vi "DAQ Loop.vi"(8 "error in":errorcluster, 10 "Queues":T1, 11 "Notifiers":T2) -> (0 "error out":errorcluster)   [LabVIEW 2015, in "DAQ.lvlib"]
uses:
  DAQ.lvlib
  support/Message Queue/Message Queue.lvlib
  TypeDefs/DAQ data.ctl
  <vilib>/ErrorRing/Error Ring.xnode
  PLC/PLC.lvlib
  support/Global names.vi
  <vilib>/Utility/error.llb/Error Cluster From Error Code.vi
  support/Message Queue/Message Cluster.ctl
  support/Notifiers/Notifiers.ctl
  Support/Notifiers/Notifiers.lvlib
  support/Message Queue/All Message Queues.ctl
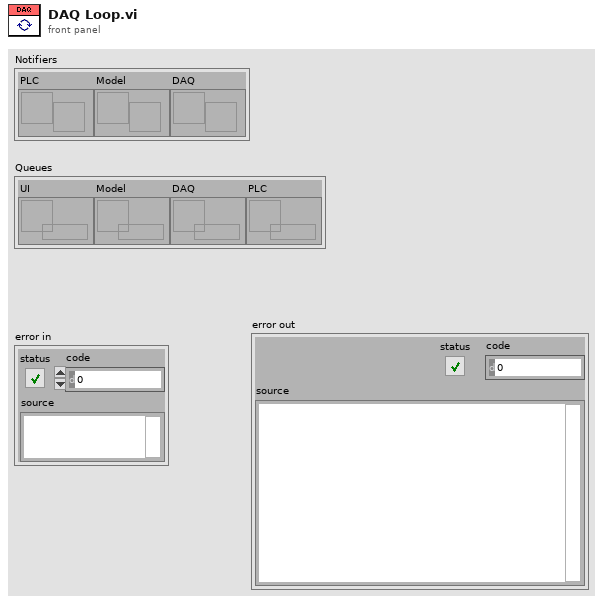
[diagram p1: front panel]
types:
  T1 = typedef "Message Queue.lvlib/All Message Queues.ctl" = cluster{"UI":refnum<queue>, "Model":refnum<queue>, "DAQ":refnum<queue>, "PLC":refnum<queue>}
  T2 = typedef "Notifiers.lvlib/Notifiers.ctl" = cluster{"PLC":refnum<notifier>, "Model":refnum<notifier>, "DAQ":refnum<notifier>}
  T3 = typedef "DAQ.lvlib/DAQ data.ctl" = cluster{"Power switch (DI)":cluster{"Channel":tag, "Data":bool}, "Dispose barrel (DI)":cluster{"Channel":tag, "Data":bool}, "Pump status (DO)":cluster{"Channel":tag, "Data":bool}, "Barrel position (AI)":cluster{"Channel":tag, "Data":dbl}}
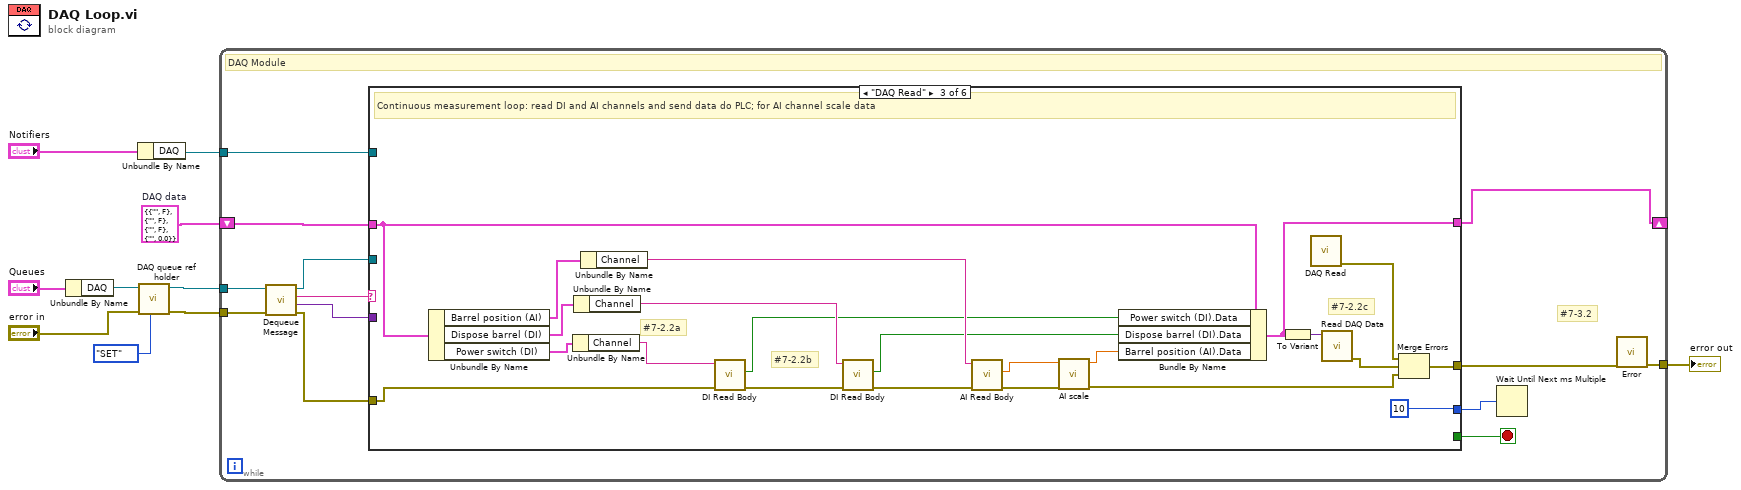
[diagram p0: block diagram]
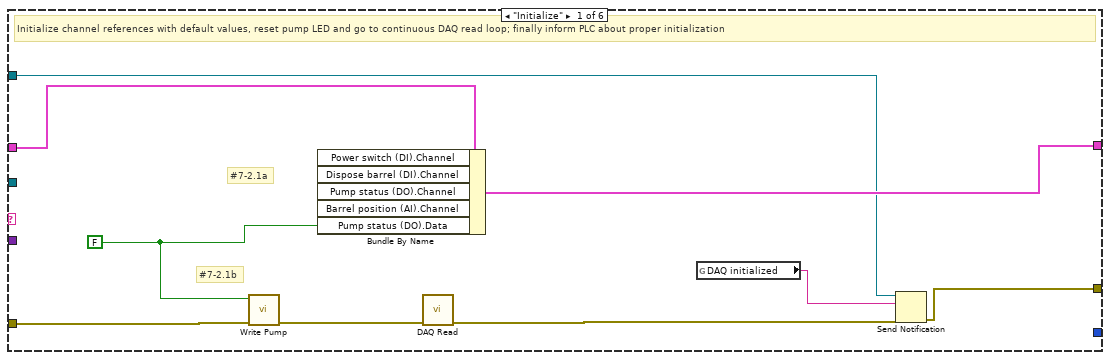
[diagram p2: hidden frame]
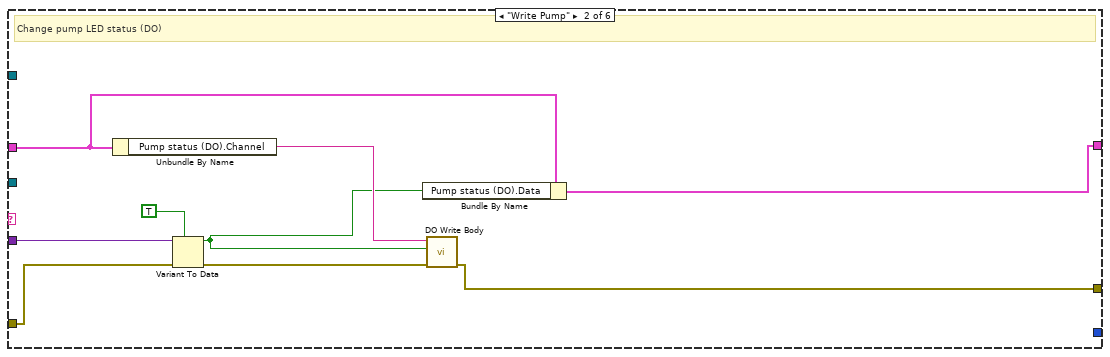
[diagram p3: hidden frame]
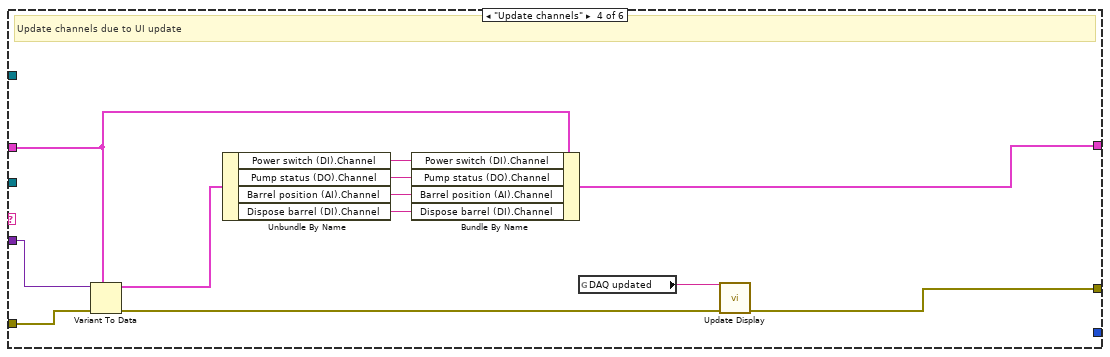
[diagram p4: hidden frame]
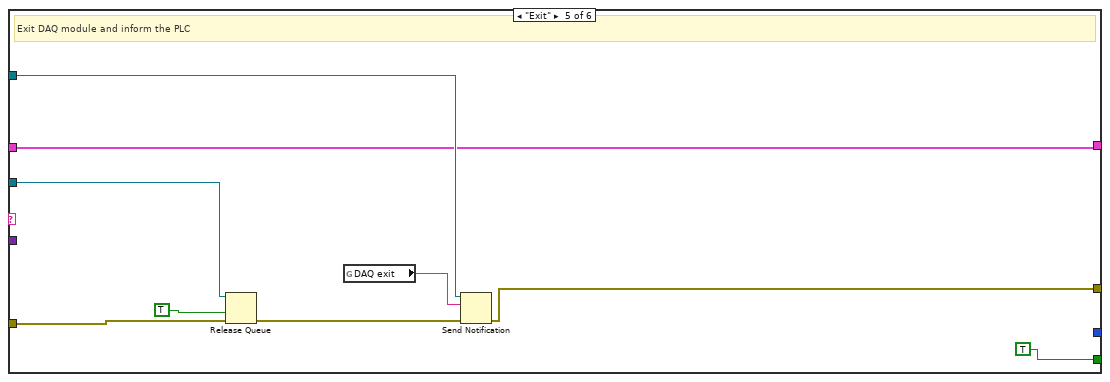
[diagram p5: hidden frame]
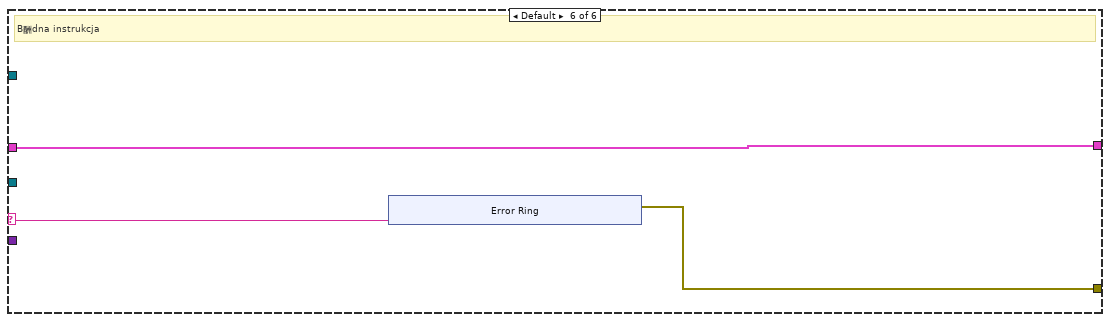
[diagram p6: hidden frame]
diagram:
  w10 = T3 {"Power switch (DI)"={"Channel"="", "Data"=FALSE}, "Dispose barrel (DI)"={"Channel"="", "Data"=FALSE}, "Pump status (DO)"={"Channel"="", "Data"=FALSE}, "Barrel position (AI)"={"Channel"="", "Data"=0.0}}  # DAQ data
  n1 = Unbundle By Name("Queues") -> ("DAQ"=w5:refnum<queue>)
  n2 = Unbundle By Name("Notifiers") -> ("DAQ"=w6:refnum<notifier>)
  n3 = call "DAQ queue ref holder.vi"("Action"=enum16{"GET", "SET"}."SET", "error in"="error in", "Message Queue In"=w5) -> ("error out"=w3:errorcluster, "Input Message Queue"=w4:refnum<queue>)  [unwired: 7 in]
  n4 = while {
    tunnel: w3 -> [w23]
    tunnel: w4 -> [w11]
    tunnel: w6 -> [w19]
    shift-right: [w18] -> _
    shift-left: w10 -> [w16]
    tunnel: [w14] -> w8
    stop <- w20 stop-if-true
    # "#7-3.2"
    # "DAQ Module"
    n5 = call "Dequeue Message.vi"("error in (no error)"=w23, "Message Queue"=w11) -> ("error out"=w22:errorcluster, "Message Data"=w21:variant, "Message"=w12:string, "dup Message Queue"=w13:refnum<queue>)  [unwired: 6 in]
    n6 = case shown="\"DAQ Read\"" w12 {
      selector: w12 -> [_ _ _ _ _ w86]
      tunnel: w22 -> [w29 w41 w56 w74 w78 _]
      tunnel: [w32 w33 w54 w66 w77 w85] -> w15
      tunnel: w21 -> [_ w40 _ w75 _ _]
      tunnel: [_ _ _ _ TRUE _] -> w20
      tunnel: w13 -> [_ _ _ _ w84 _]
      tunnel: w19 -> [w27 _ _ _ w83 _]
      tunnel: w16 -> [w31 w37 w61 w73 w79 w87]
      tunnel: [w30 w39 w58 w68 w79 w87] -> w18
      tunnel: [_ _ u32 10 ("millisecond multiple") _ _ _] -> w17
      frame "Initialize" {
        w24 = FALSE ("Pump status (DO).Data")
        # "#7-2.1b"
        # "#7-2.1a"
        # "Initialize channel references with default values, reset pump LED and go to continuous DAQ read loop; finally inform PLC about proper initialization"
        n7 = call "Write Pump.vi"("error in"=w29, "Pump state"=w24) -> ("error out"=w28:errorcluster)  [unwired: 9 in]
        n8 = Bundle By Name(cluster=w31, "Pump status (DO).Data"=w24) -> (w30:T3)  [unwired: 4 in]
        n9 = call "DAQ Read.vi"("error in"=w28) -> ("error out"=w26:errorcluster)  [unwired: 10 in]
        n10 = global read "Global names.vi" "DAQ initialized"() -> (w25:string)
        n11 = Send Notification(notification=w25, notifier=w27, error in (no error)=w26) -> (error out=w32:errorcluster)  [unwired: 1 out]
      }
      frame "Write Pump" {
        # "Change pump LED status (DO)"
        n12 = Unbundle By Name(w37) -> ("Pump status (DO).Channel"=w38:tag)
        n13 = Variant To Data(error in=w41, type=TRUE, Variant=w40) -> (data=w35:bool, error out=w34:errorcluster)
        n14 = Bundle By Name(cluster=w37, "Pump status (DO).Data"=w35) -> (w39:T3)
        n15 = call "DO Write Body.vi"("error in"=w34, "data"=w35, "Channel"=w38) -> ("error out"=w33:errorcluster)  [unwired: 6 in]
      }
      frame "DAQ Read" {
        # "#7-2.2c"
        # "#7-2.2b"
        # "#7-2.2a"
        # "Continuous measurement loop: read DI and AI channels and send data do PLC; for AI channel scale data"
        n16 = Unbundle By Name(w61) -> ("Barrel position (AI)"=w50:cluster{"Channel":tag, "Data":dbl}, "Dispose barrel (DI)"=w49:cluster{"Channel":tag, "Data":bool}, "Power switch (DI)"=w48:cluster{"Channel":tag, "Data":bool})
        n17 = Unbundle By Name(w48) -> ("Channel"=w45:tag)
        n18 = Unbundle By Name(w49) -> ("Channel"=w46:tag)
        n19 = Unbundle By Name(w50) -> ("Channel"=w47:tag)
        n20 = call "DI Read Body.vi"("error in"=w56, "Channel"=w45) -> ("error out"=w63:errorcluster, "data"=w44:bool)  [unwired: 6 in]
        n21 = call "DI Read Body.vi"("error in"=w63, "Channel"=w46) -> ("error out"=w62:errorcluster, "data"=w43:bool)  [unwired: 6 in]
        n22 = call "AI Read Body.vi"("error in"=w62, "Channel"=w47) -> ("error out"=w55:errorcluster, "data"=w51:dbl)  [unwired: 6 in]
        n23 = call "AI scale.vi"("error in"=w55, "Data in"=w51) -> ("error out"=w52:errorcluster, "Data out"=w60:dbl)  [unwired: 8 in]
        n24 = Bundle By Name(cluster=w61, "Power switch (DI).Data"=w44, "Dispose barrel (DI).Data"=w43, "Barrel position (AI).Data"=w60) -> (w58:T3)
        n25 = To Variant(anything=w58) -> (Variant=w57:variant)
        n26 = call "DAQ Read.vi"() -> ("error out"=w42:errorcluster)  [unwired: 11 in]
        n27 = call "Read DAQ Data.vi"("Message Data"=w57) -> ("error out"=w53:errorcluster)  [unwired: 10 in]
        n28 = Merge Errors(w42, w53, w52) -> (w54:errorcluster)
      }
      frame "Update channels" {
        # "Update channels due to UI update"
        n29 = Variant To Data(error in=w74, type=w73, Variant=w75) -> (data=w65:T3, error out=w67:errorcluster)
        n30 = Unbundle By Name(w65) -> ("Power switch (DI).Channel"=w72:tag, "Pump status (DO).Channel"=w71:tag, "Barrel position (AI).Channel"=w70:tag, "Dispose barrel (DI).Channel"=w69:tag)
        n31 = Bundle By Name(cluster=w73, "Power switch (DI).Channel"=w72, "Pump status (DO).Channel"=w71, "Barrel position (AI).Channel"=w70, "Dispose barrel (DI).Channel"=w69) -> (w68:T3)
        n32 = global read "Global names.vi" "DAQ updated"() -> (w64:string)
        n33 = call "Update Display.vi"("error in"=w67, "Message string"=w64) -> ("error out"=w66:errorcluster)  [unwired: 9 in]
      }
      frame "Exit" {
        # "Exit DAQ module and inform the PLC"
        n34 = Release Queue(queue=w84, force destroy? (F)=TRUE, error in (no error)=w78) -> (error out=w82:errorcluster)  [unwired: 2 out]
        n35 = global read "Global names.vi" "DAQ exit"() -> (w76:string)
        n36 = Send Notification(notification=w76, notifier=w83, error in (no error)=w82) -> (error out=w77:errorcluster)  [unwired: 1 out]
      }
      frame Default {
        # "B酬dna instrukcja"
        n37 = xnode "Error Ring"("parameter 0"=w86) -> ("error out"=w85:errorcluster)
      }
    }
    n38 = Wait Until Next ms Multiple(millisecond multiple=w17) -> ()  [unwired: 1 out]
    n39 = call "Error.vi"("error in"=w15) -> ("error out"=w14:errorcluster)  [unwired: 10 in]
  }
  "error out" <- w8
